vi "Instance FG.vi"(8 "error in (no error)":errorcluster, 11 "picoG in":refnum<class "picoG.lvclass">) -> (0 "error out":errorcluster, 3 "picoG out":refnum<class "picoG.lvclass">)   [LabVIEW 2020, in "PicoG-App.lvlib" / "picoG.lvclass"]
uses:
  picoG.lvclass
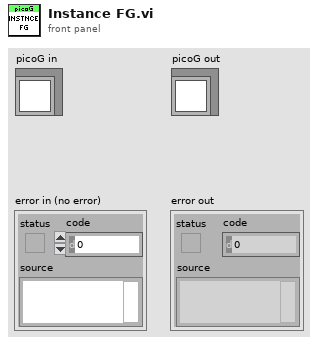
[diagram p1: front panel]
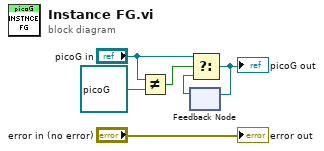
[diagram p0: block diagram]
diagram:
  n1 = Not Equal?(x="picoG in", y=refnum<class "picoG.lvclass"> refnum ("App in")) -> (x != y?=w1:bool)
  n2 = feedback #1() -> (w4:refnum<class "picoG.lvclass">)  [unwired: 1 in]
  n3 = Select(t="picoG in", s=w1, f=w4) -> (s? t:f=w5:refnum<class "picoG.lvclass">)
  "picoG out" <- w5
  n4 = feedback-in #1(w5) -> ()
  "error out" <- "error in (no error)"
